vi "PI Start WG.vi"(0 "System no.":i32=1 min=1 max=4 step=1, 1 "axis":string="xy", 2 "Generator":i8 min=0 max=2 step=1, 3 "Init DDL":i8 min=0 max=3 step=1, 4 "increment":i8 min=0 max=3 step=1, 5 "error in":errorcluster, 14 "saved data":i8 min=0 max=3 step=1) -> (19 "error out":errorcluster)   [LabVIEW 2013]
doc: "Sends command with or without trailing linefeed to selected system. \n\nValid for C-843, C-843.PM, C-844, C-848, C-865, C-880, C-880K005, E-516, E-710, E-816, F-206, M-8X0"
panel:
  out "String":string
  # "This vi sends a string w/o linefeed via the GPIB interface."
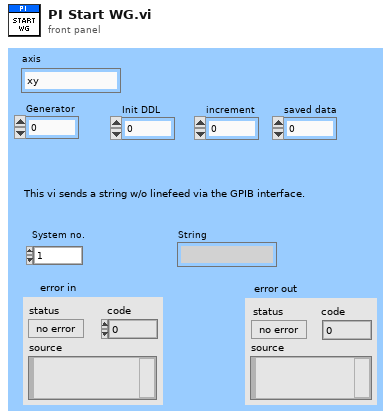
[diagram p1: front panel]
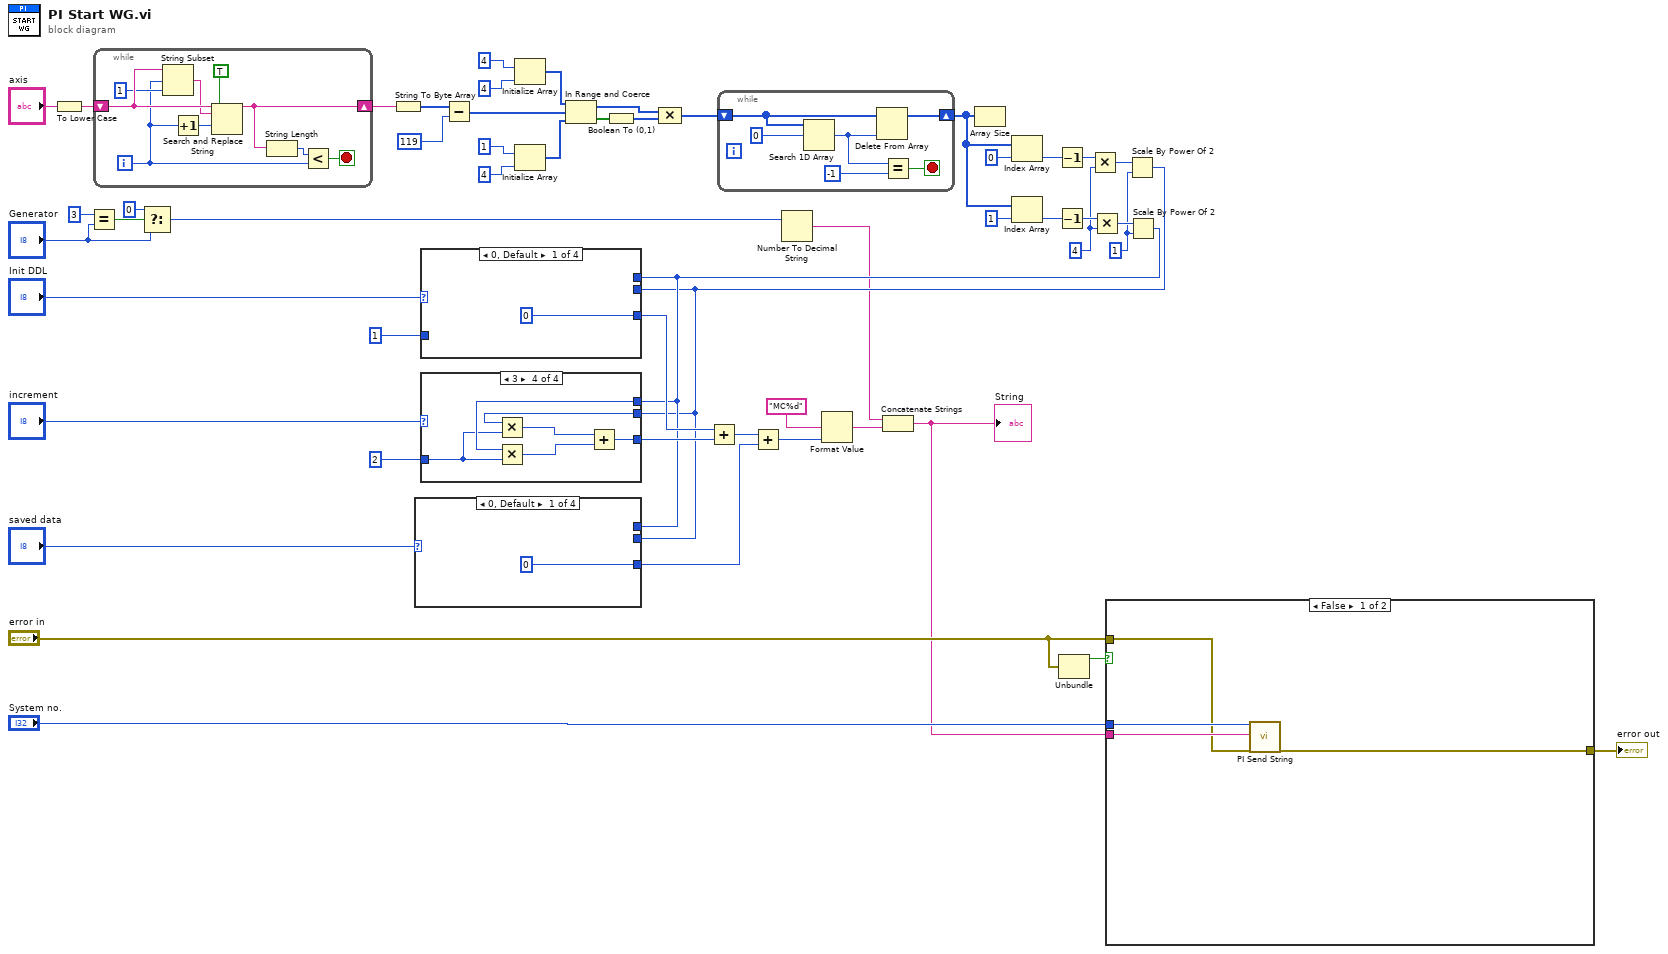
[diagram p0: block diagram]
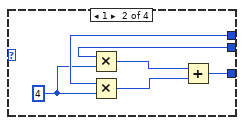
[diagram p2: hidden frame]
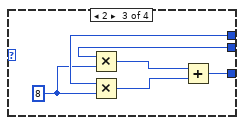
[diagram p3: hidden frame]
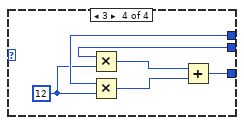
[diagram p4: hidden frame]
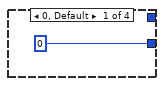
[diagram p5: hidden frame]
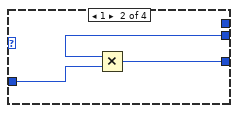
[diagram p6: hidden frame]
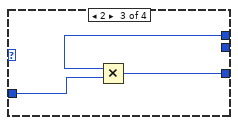
[diagram p7: hidden frame]
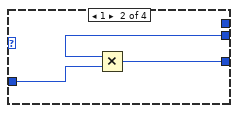
[diagram p8: hidden frame]
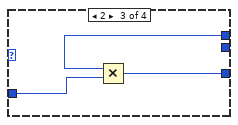
[diagram p9: hidden frame]
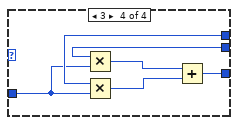
[diagram p10: hidden frame]
diagram:
  w23 = 1
  w24 = 4
  n1 = To Lower Case(string="axis") -> (all lower case string=w35:string)
  n2 = Equal?(x=3, y="Generator") -> (x = y?=w7:bool)
  n3 = while {
    shift-right: [w57] -> w40
    shift-left: w35 -> [w61]
    i -> [w53]
    stop <- w56 stop-if-true
    n4 = String Subset(string=w61, offset (0)=w53, length (rest)=1) -> (substring=w59:string)
    n5 = Increment(x=w53) -> (x+1=w54:i32)
    n6 = Search and Replace String(replace all?=TRUE, input string=w61, search string=w59, offset=w54) -> (result string=w57:string)  [unwired: 4 in, 3 out]
    n7 = String Length(string=w57) -> (length=w55:i32)
    n8 = Less?(x=w55, y=w53) -> (x < y?=w56:bool)
  }
  n9 = Select(t=0, s=w7, f="Generator") -> (s? t:f=w5:i32)
  n10 = String To Byte Array(string=w40) -> (unsigned byte array=w42:u8[])
  n11 = Subtract(x=w42, y=119) -> (x-y=w39:i32[])
  n12 = Initialize Array(4, 4) -> (w47:i32[])
  n13 = Initialize Array(1, 4) -> (w44:i32[])
  n14 = In Range and Coerce(upper limit=w47, x=w39, lower limit=w44) -> (coerced(x)=w36:i32[], In Range?=w43:bool[])
  n15 = Boolean To (0,1)(Boolean=w43) -> (0, 1=w37:i16[])
  n16 = Compound Arithmetic op=MULTIPLY(w36, w37) -> (w38:i32[])
  n17 = while {
    shift-right: [w64] -> w32
    shift-left: w38 -> [w62]
    stop <- w65 stop-if-true
    n18 = Search 1D Array(1D array=w62, element=0) -> (index of element=w66:i32)  [unwired: 1 in]
    n19 = Delete From Array(array=w62, index=w66) -> (array with subset deleted=w64:i32[])  [unwired: 1 in, 1 out]
    n20 = Equal?(x=w66, y=-1) -> (x = y?=w65:bool)
  }
  n21 = Number To Decimal String(number=w5) -> (decimal integer string=w8:string)  [unwired: 1 in]
  n22 = Array Size(array=w32) -> ()  [unwired: 1 out]
  n23 = Index Array(array=w32, index=0) -> (element=w31:i32)
  n24 = Index Array(array=w32, index=1) -> (element=w30:i32)
  n25 = Decrement(x=w31) -> (x-1=w28:i32)
  n26 = Decrement(x=w30) -> (x-1=w27:i32)
  n27 = Unbundle("error in") -> ("status"=w52:bool)  [unwired: 2 out]
  n28 = Multiply(x=w28, y=w24) -> (x*y=w26:i32)
  n29 = Multiply(x=w27, y=w24) -> (x*y=w25:i32)
  n30 = Scale By Power Of 2(n=w26, x=w23) -> (x*2^n=w14:i32)
  n31 = Scale By Power Of 2(n=w25, x=w23) -> (x*2^n=w15:i32)
  n32 = case shown="0, Default" "saved data" {
    tunnel: w14 -> [_ w70 w76 w82]
    tunnel: [0 w73 w79 w85] -> w12
    tunnel: w15 -> [_ w74 w80 w86]
    frame 0, Default {
    }
    frame 1 {
      w69 = 4
      n33 = Multiply(x=w70, y=w69) -> (x*y=w71:i32)
      n34 = Multiply(x=w74, y=w69) -> (x*y=w72:i32)
      n35 = Add(x=w71, y=w72) -> (x+y=w73:i32)
    }
    frame 2 {
      w75 = 8
      n36 = Multiply(x=w76, y=w75) -> (x*y=w77:i32)
      n37 = Multiply(x=w80, y=w75) -> (x*y=w78:i32)
      n38 = Add(x=w77, y=w78) -> (x+y=w79:i32)
    }
    frame 3 {
      w81 = 12
      n39 = Multiply(x=w82, y=w81) -> (x*y=w83:i32)
      n40 = Multiply(x=w86, y=w81) -> (x*y=w84:i32)
      n41 = Add(x=w83, y=w84) -> (x+y=w85:i32)
    }
  }
  n42 = case shown="0, Default" "Init DDL" {
    tunnel: w14 -> [_ w90 _ w94]
    tunnel: [0 w89 w93 w97] -> w19
    tunnel: w15 -> [_ _ w91 w99]
    tunnel: 1 -> [_ w88 w92 w98]
    frame 0, Default {
    }
    frame 1 {
      n43 = Multiply(x=w90, y=w88) -> (x*y=w89:i32)
    }
    frame 2 {
      n44 = Multiply(x=w91, y=w92) -> (x*y=w93:i32)
    }
    frame 3 {
      n45 = Multiply(x=w94, y=w98) -> (x*y=w95:i32)
      n46 = Multiply(x=w99, y=w98) -> (x*y=w96:i32)
      n47 = Add(x=w95, y=w96) -> (x+y=w97:i32)
    }
  }
  n48 = case shown="3" "increment" {
    tunnel: w14 -> [_ w103 _ w107]
    tunnel: [0 w102 w106 w110] -> w18
    tunnel: w15 -> [_ _ w104 w112]
    tunnel: 2 -> [_ w101 w105 w111]
    frame 0, Default {
    }
    frame 1 {
      n49 = Multiply(x=w103, y=w101) -> (x*y=w102:i32)
    }
    frame 2 {
      n50 = Multiply(x=w104, y=w105) -> (x*y=w106:i32)
    }
    frame 3 {
      n51 = Multiply(x=w107, y=w111) -> (x*y=w108:i32)
      n52 = Multiply(x=w112, y=w111) -> (x*y=w109:i32)
      n53 = Add(x=w108, y=w109) -> (x+y=w110:i32)
    }
  }
  n54 = Add(x=w19, y=w18) -> (x+y=w13:i32)
  n55 = Add(x=w13, y=w12) -> (x+y=w11:i32)
  n56 = Format Value(format string="MC%d", value (0)=w11) -> (output string=w9:string)  [unwired: 1 in]
  n57 = Concatenate Strings(w8, w9) -> (w1:string)
  "String" <- w1
  n58 = case shown="False" w52 {
    tunnel: [w113 w117] -> w50
    tunnel: "error in" -> [w114 w117]
    tunnel: w1 -> [w115 _]
    tunnel: "System no." -> [w116 _]
    frame False {
      n59 = call "PI Send String.vi"("System no."=w116, "String to send"=w115, "error in"=w114) -> ("error out"=w113:errorcluster)  [unwired: 16 in]
    }
    frame True {
      # "Error!"
    }
  }
  "error out" <- w50
